vi "f2+g2u.vi"(0 "x3_":dbl, 1 "x4_":dbl, 2 "u":dbl) -> (20 "f2+g2u":dbl)   [LabVIEW 2014]
uses:
  <vilib>/Simulation/Implementation/Shared/SIMSCR Execution Mode.ctl
  <vilib>/Simulation/Scripting/Companion Diagram/SimConfigNode/SimParams.ctl
  <vilib>/Simulation/Scripting/Companion Diagram/SimConfigNode/_simSolvers.ctl
  <vilib>/Simulation/Param Hierarchy/Typedefs/SIMPH Param Control Actions.ctl
  <vilib>/Simulation/Implementation/Shared/NILVSim_ParamChanged.vi
  <vilib>/Simulation/Implementation/Shared/NILVSIM_BeginStep.vi
  <vilib>/Simulation/SignalArithmetic/Implementation/NILVSim Gain.llb/SIM Gain (scalar).vi
  <vilib>/Simulation/Implementation/Shared/NILVSim_Manager.vi
  <vilib>/Utility/error.llb/Clear Errors.vi
  <vilib>/Simulation/Implementation/Shared/NILVSim_FinalizeModel.vi
  <vilib>/Simulation/Implementation/Shared/SIM Unbundle Sim Info.vi
  <vilib>/Simulation/Implementation/Shared/SIMSH Read Queue.vi
  <vilib>/Simulation/Implementation/Shared/NILVSim_Initialize.vi
  <vilib>/Simulation/Utility/Implementation/NILVSim Get Time and IsAcceptedStep.vi
  <vilib>/Simulation/Implementation/Shared/NILVSim_GetModelError.vi
  <vilib>/Simulation/Implementation/Shared/SIM SimErrorHandler.vi
  <vilib>/Simulation/Implementation/Shared/SIM Bundle Sim Info.vi
  <vilib>/Simulation/Scripting/Companion Diagram/SimConfigNode/SimDog.xnode
  <vilib>/Simulation/Implementation/XNodeFramework/SimXNode/SimX.xnode
  <vilib>/Simulation/Implementation/Shared/NI_SIM_Implementation.lvlib
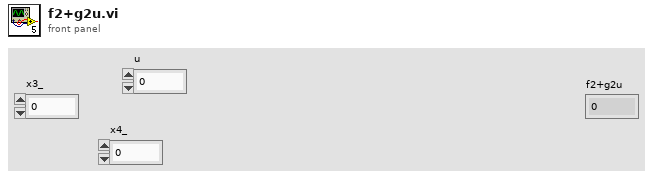
[diagram p1: front panel]
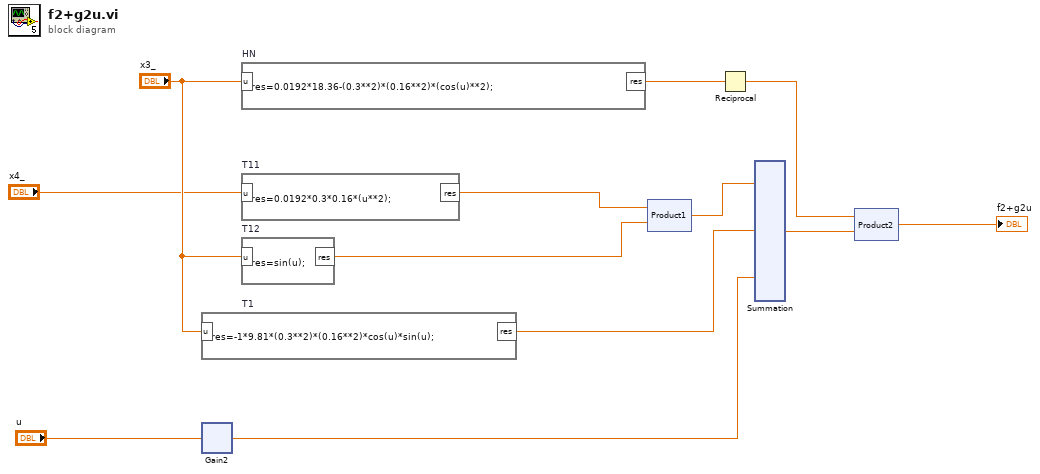
[diagram p0: block diagram]
diagram:
  n1 = formula code="res=-1*9.81*(0.3**2)*(0.16**2)*cos(u)*sin(u);" "T1"("u"="x3_") -> ("res"=w5:dbl)
  n2 = xnode "Gain2"("input"="u") -> ("output"=w4:dbl)  [unwired: 3 in]
  n3 = formula code="res=0.0192*18.36-(0.3**2)*(0.16**2)*(cos(u)**2);" "HN"("u"="x3_") -> ("res"=w11:dbl)
  n4 = formula code="res=0.0192*0.3*0.16*(u**2);" "T11"("u"="x4_") -> ("res"=w8:dbl)
  n5 = formula code="res=sin(u);" "T12"("u"="x3_") -> ("res"=w7:dbl)
  n6 = xnode "Product1"("Operand1"=w8, "Operand2"=w7) -> ("Result"=w6:dbl)
  n7 = Reciprocal ("Math\\nFunction")(x=w11) -> (1/x=w3:dbl)
  n8 = xnode ("Summation")("Operand1"=w6, "Operand2"=w5, "Operand3"=w4) -> ("Result"=w2:dbl)
  n9 = xnode ("Product2")("Operand1"=w3, "Operand2"=w2) -> ("Result"=→"f2+g2u":dbl)
